vi "Write Payload.vi"(10 "Payload":string, 11 "GDSII.DataType.String in":refnum<class "GDSII.DataType.String.lvclass">) -> (3 "GDSII.DataType.String out":refnum<class "GDSII.DataType.String.lvclass">)   [LabVIEW 2019, in "GDSII.DataType.String.lvclass"]
uses:
  GDSII.DataType.String.lvclass
  GDSII.DataType.String.lvclass/GDSII.DataType.String.ctl
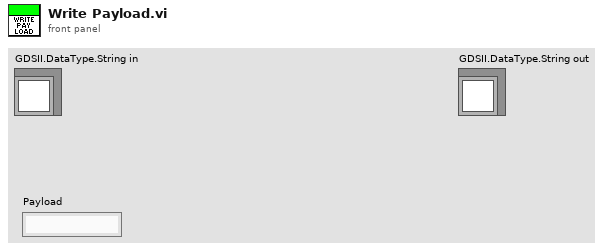
[diagram p1: front panel]
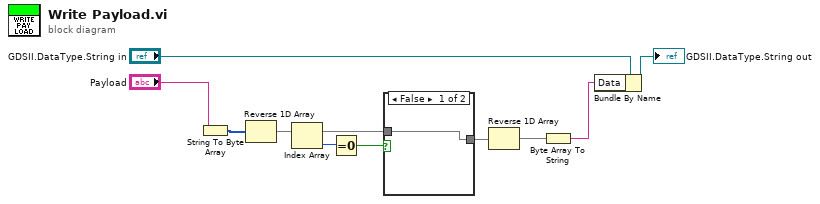
[diagram p0: block diagram]
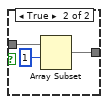
[diagram p2: hidden frame]
diagram:
  n1 = String To Byte Array(string="Payload") -> (unsigned byte array=w8:u8[])
  n2 = Reverse 1D Array(array=w8) -> (reversed array=w5:u8[])
  n3 = Index Array(array=w5) -> (element=w7:u8)  [unwired: 1 in]
  n4 = Equal To 0?(x=w7) -> (x = 0?=w6:bool)
  n5 = case shown="False" w6 {
    tunnel: w5 -> [w11 w14]
    tunnel: [w11 w12] -> w4
    frame False {
    }
    frame True {
      n6 = Array Subset(array=w14, index=1) -> (w12:u8[])  [unwired: 1 in]
    }
  }
  n7 = Reverse 1D Array(array=w4) -> (reversed array=w3:u8[])
  n8 = Byte Array To String(unsigned byte array=w3) -> (string=w1:string)
  n9 = Bundle By Name(cluster="GDSII.DataType.String in", "Data"=w1) -> (→"GDSII.DataType.String out":refnum<class "GDSII.DataType.String.lvclass">)
